vi "NT Write Name Cache.vi"(8 "Field Value In":T1, 11 "Name":string) -> (0 "Field Value Out":T1)   [LabVIEW 2017]
uses:
  <vilib>/Rock Robotics/Network Tables/Field Data.ctl
  <vilib>/Rock Robotics/Network Tables/Field Type.ctl
  <vilib>/Rock Robotics/Network Tables/Sequence.ctl
  <vilib>/Rock Robotics/Network Tables/Create Actual Table Name.vi
  <vilib>/Rock Robotics/Network Tables/Manage Dirty Field ID List.vi
  <vilib>/Rock Robotics/Network Tables/NT Globals.vi
  <vilib>/Rock Robotics/Network Tables/Update Other Clients.vi
  <vilib>/Rock Robotics/Network Tables/Build Entry Assign Buffer.vi
  <vilib>/Rock Robotics/Network Tables/Field Data Manager.vi
  <vilib>/Rock Robotics/Network Tables/Usage Statistics.vi
  <vilib>/Rock Robotics/Network Tables/Table Manager.vi
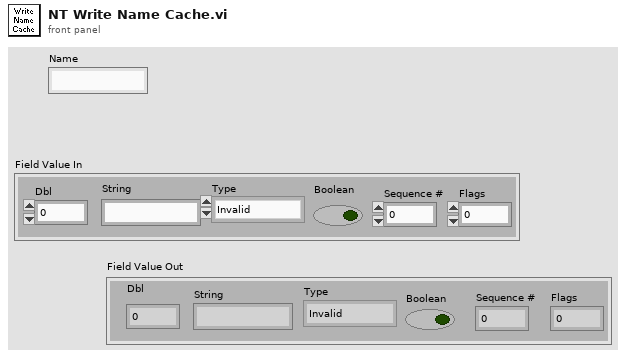
[diagram p1: front panel]
types:
  T1 = typedef "Field Data.ctl" = cluster{"Dbl":dbl, "String":string, "Type":T2, "Boolean":bool, "Sequence #":T3, "Flags":u8}
  T2 = typedef "Field Type.ctl" = enum8{"Invalid", "Bool", "Numeric", "String", "Raw", "Boolean Array", "Numeric Array", "String Array", "RPC"}
  T3 = typedef "Sequence.ctl" = u16
  T4 = typedef "Field ID.ctl" = i32
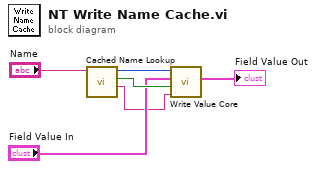
[diagram p0: block diagram]
diagram:
  n1 = call <vilib>:"Cached Name Lookup.vi"("Name"="Name") -> ("Full Name"=w1:string, "Success"=w6:bool, "Entry ID"=w4:T4)  [unwired: 8 in]
  n2 = call <vilib>:"Write Value Core.vi"("Name"=w1, "Existing"=w6, "Field Value"="Field Value In", "Field ID"=w4) -> ("Field Value Out"=→"Field Value Out":T1)  [unwired: 7 in]
